vi "Eliminated.vi"(6 "Column":i32, 8 "Row":i32, 9 "Killer Index":i32, 10 "Team Index":i32, 11 "Atom in":refnum<class "Atom.lvclass">) -> (3 "Atom out":refnum<class "Atom.lvclass">)   [LabVIEW 2017, in "Atom.lvclass"]
uses:
  Atom.lvclass
  Square/Square.lvclass
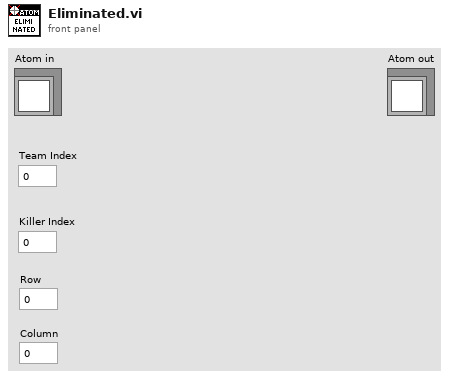
[diagram p1: front panel]
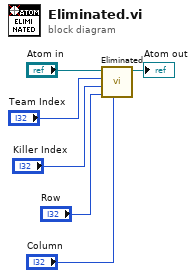
[diagram p0: block diagram]
diagram:
  n1 = call-parent "Eliminated.vi"("Column"="Column", "Row"="Row", "Killer Index"="Killer Index", "Team Index"="Team Index", "Square in"="Atom in") -> ("Square out"=→"Atom out":refnum<class "Atom.lvclass">)  [unwired: 6 in]
